vi "IMAQ FPGA Camera Link Pixel Packer U8x2.vi"(8 "Input Valid":bool, 9 "Frame Valid In":bool, 10 "Line Valid In":bool, 11 "Pixels In":u8[](array[numeric])=[0, 0]) -> (0 "Output Valid":bool, 1 "Frame Valid Out":bool, 2 "Line Valid Out":bool, 3 "Pixel Bus x8 Out":cluster{"Pixels":u8[], "DV":bool[]})   [LabVIEW 2017]
doc: "The Pixel Packer combines pixels from different cycles to create a Pixel Bus with 8 adjacent pixels. The DV flag in the Pixel Bus x8 Out indicates if the corresponding pixel is valid in case there are cameras with a width that is not a multiple of 8."
uses:
  <vilib>/visionFPGA/Basics/Camera Link Acquisition/Controls/IMAQ FPGA Camera Link Pixel Packer State.ctl
  <vilib>/visionFPGA/NI_VDM_FPGA_Basics.lvlib
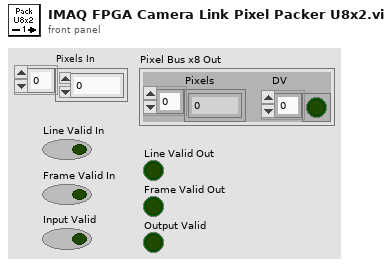
[diagram p1: front panel]
types:
  T1 = typedef "IMAQ FPGA Camera Link Pixel Packer State.ctl" = enum16{"Wait to Pack", "Pack", "Add EOL", "Check EOI"}
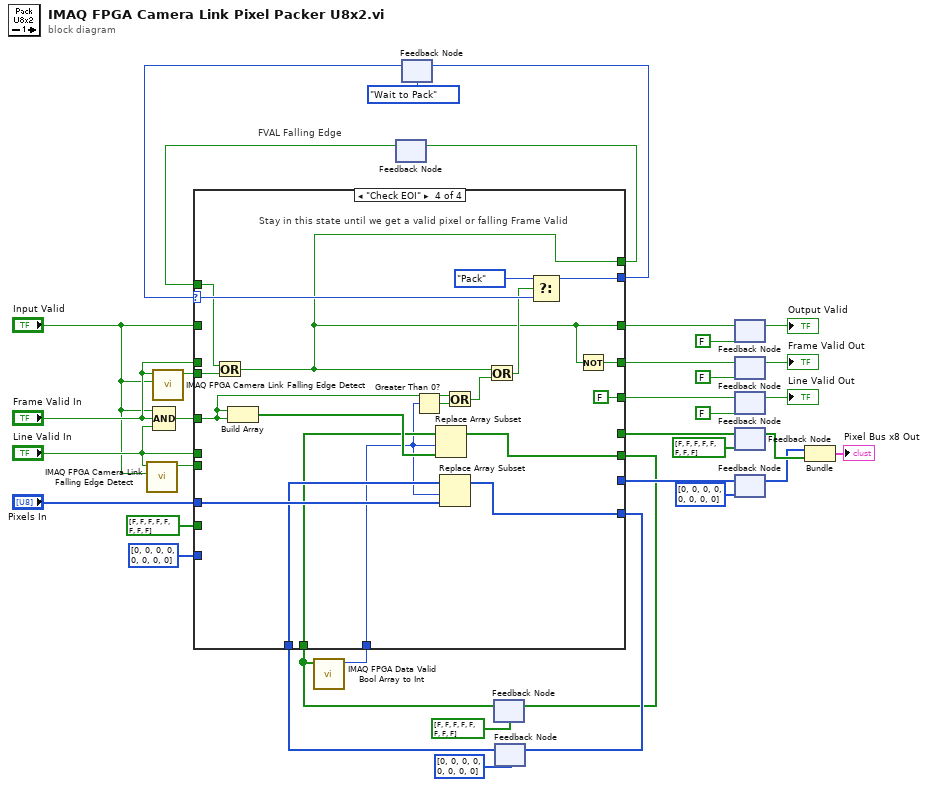
[diagram p0: block diagram]
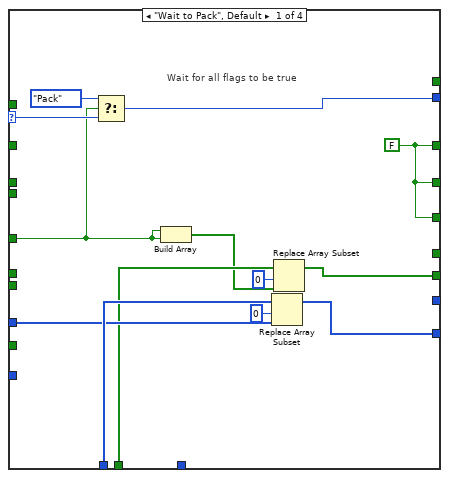
[diagram p2: hidden frame]
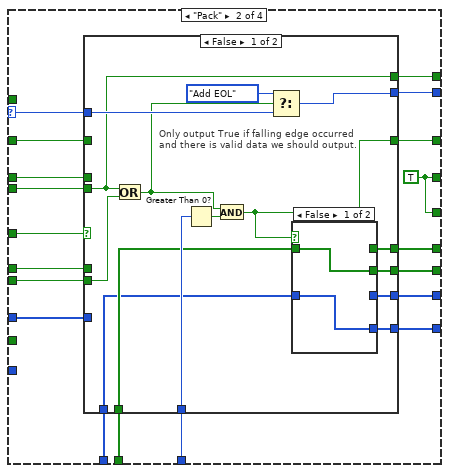
[diagram p3: hidden frame]
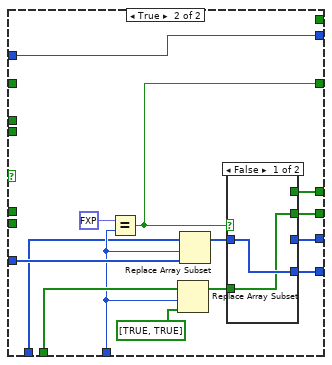
[diagram p5: hidden frame]
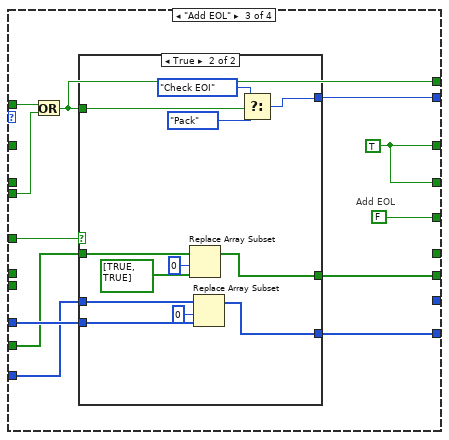
[diagram p7: hidden frame]
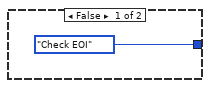
[diagram p8: hidden frame]
diagram:
  # "FVAL Falling Edge"
  n1 = call <vilib>:"IMAQ FPGA Camera Link Falling Edge Detect.vi"("Input Valid"="Input Valid", "Input"="Line Valid In") -> ("Falling Edge"=w7:bool)  [unwired: 9 in]
  n2 = call <vilib>:"IMAQ FPGA Camera Link Falling Edge Detect.vi"("Input Valid"="Input Valid", "Input"="Frame Valid In") -> ("Falling Edge"=w10:bool)  [unwired: 9 in]
  n3 = Compound Arithmetic op=AND("Input Valid", "Frame Valid In", "Line Valid In") -> (w16:bool)
  n4 = feedback #1() -> (w1:bool)  [unwired: 1 in]
  n5 = feedback #2(IMAQ_FPGA_Camera_Link_Pixel_Packer_State."Wait to Pack" ("Enum")) -> (w18:T1)
  n6 = feedback #3(bool[] [FALSE, FALSE, FALSE, FALSE, FALSE, FALSE, FALSE, FALSE]) -> (w4:bool[])
  n7 = call <vilib>:"IMAQ FPGA Data Valid Bool Array to Int.vi"("DV In"=w4) -> ("Sum DV Out"=w3:u8)  [unwired: 10 in]
  n8 = feedback #4(u8[] [0, 0, 0, 0, 0, 0, 0, 0] ("Pixels")) -> (w30:u8[])
  n9 = case shown="\"Check EOI\"" w18 {
    selector: w18 -> [w50 w68 _ w150]
    tunnel: w4 -> [w44 w56 _ w137]
    tunnel: w30 -> [w48 w67 _ w138]
    tunnel: [_ w64 _ _] -> w29
    tunnel: [_ w63 _ _] -> w22
    tunnel: [w38 w62 w118 w141] -> w36
    tunnel: [w38 w53 w118 w140] -> w20
    tunnel: [w38 w53 FALSE FALSE ("Frame Valid In")] -> w19
    tunnel: "Frame Valid In" -> [_ w60 _ _]
    tunnel: "Line Valid In" -> [_ w61 _ _]
    tunnel: "Input Valid" -> [_ w59 _ _]
    tunnel: w16 -> [w40 w69 w117 w134]
    tunnel: "Pixels In" -> [w46 w57 w114 w148]
    tunnel: [w45 w66 w113 w146] -> w14
    tunnel: [w42 w65 w115 w147] -> w13
    tunnel: [w41 w58 w116 w149] -> w12
    tunnel: w10 -> [_ w55 w108 w142]
    tunnel: w7 -> [_ w54 _ _]
    tunnel: u8[] [0, 0, 0, 0, 0, 0, 0, 0] ("Pixels") -> [_ _ w111 _]
    tunnel: bool[] [FALSE, FALSE, FALSE, FALSE, FALSE, FALSE, FALSE, FALSE] -> [_ _ w110 _]
    tunnel: w3 -> [_ w52 _ w136]
    tunnel: [_ w51 w107 w141] -> w2
    tunnel: w1 -> [_ _ w109 w143]
    frame "Wait to Pack", Default {
      w38 = FALSE
      # "Wait for all flags to be true"
      n10 = Select(t=IMAQ_FPGA_Camera_Link_Pixel_Packer_State."Pack", s=w40, f=w50) -> (s? t:f=w41:T1)
      n11 = Build Array(w40, w40) -> (w39:bool[])
      n12 = Replace Array Subset(array=w48, new element=w46, index=0) -> (w45:u8[])
      n13 = Replace Array Subset(array=w44, new element=w39, index=0) -> (w42:bool[])
    }
    frame "Pack" {
      w53 = TRUE ("Frame Valid In")
      n14 = case shown="False" w69 {
        tunnel: w68 -> [w83 w101]
        tunnel: [w81 w101] -> w58
        tunnel: w67 -> [w76 w94]
        tunnel: [w71 w91] -> w66
        tunnel: w56 -> [w77 w102]
        tunnel: [w72 w97] -> w65
        tunnel: [w74 w92] -> w64
        tunnel: [w75 w98] -> w63
        tunnel: w59 -> [_ _]
        tunnel: [w73 w100] -> w62
        tunnel: w60 -> [_ _]
        tunnel: w61 -> [_ _]
        tunnel: w55 -> [w70 _]
        tunnel: w54 -> [w84 _]
        tunnel: w52 -> [w80 w95]
        tunnel: w57 -> [_ w96]
        tunnel: [w70 _] -> w51
        frame False {
          # "Only output True if falling edge occurred and there is valid data we should output."
          n15 = Or(x=w70, y=w84) -> (x .or. y?=w78:bool)
          n16 = Greater Than 0?(x=w80) -> (x > 0?=w79:bool)
          n17 = And(x=w78, y=w79) -> (x .and. y?=w73:bool)
          n18 = Select(t=IMAQ_FPGA_Camera_Link_Pixel_Packer_State."Add EOL", s=w78, f=w83) -> (s? t:f=w81:T1)
          n19 = case shown="False" w73 {
            tunnel: w77 -> [w86 w88]
            tunnel: w76 -> [w85 w87]
            tunnel: [_ w88] -> w75
            tunnel: [_ w87] -> w74
            tunnel: [w86 _] -> w72
            tunnel: [w85 _] -> w71
            frame False {
            }
            frame True {
            }
          }
        }
        frame True {
          n20 = Equal?(x=fxp<+,4,4> 6.0, y=w95) -> (x = y?=w100:bool)
          n21 = Replace Array Subset(array=w102, new element=bool[] [TRUE, TRUE], index=w95) -> (w99:bool[])
          n22 = Replace Array Subset(array=w94, new element=w96, index=w95) -> (w93:u8[])
          n23 = case shown="False" w100 {
            tunnel: w99 -> [w103 w106]
            tunnel: [_ w106] -> w98
            tunnel: [w103 _] -> w97
            tunnel: w93 -> [w104 w105]
            tunnel: [_ w105] -> w92
            tunnel: [w104 _] -> w91
            frame False {
            }
            frame True {
            }
          }
        }
      }
    }
    frame "Add EOL" {
      w118 = TRUE
      # "Add EOL"
      n24 = Or(x=w109, y=w108) -> (x .or. y?=w107:bool)
      n25 = case shown="True" w117 {
        tunnel: [IMAQ_FPGA_Camera_Link_Pixel_Packer_State."Check EOI" ("Enum") w120] -> w116
        tunnel: w110 -> [_ w131]
        tunnel: [_ w130] -> w115
        tunnel: w111 -> [_ w129]
        tunnel: w114 -> [_ w128]
        tunnel: [_ w126] -> w113
        tunnel: w107 -> [_ w121]
        frame False {
        }
        frame True {
          n26 = Replace Array Subset(array=w131, new element=bool[] [TRUE, TRUE], index=0) -> (w130:bool[])
          n27 = Replace Array Subset(array=w129, new element=w128, index=0) -> (w126:u8[])
          n28 = Select(t=IMAQ_FPGA_Camera_Link_Pixel_Packer_State."Check EOI" ("Enum"), s=w121, f=IMAQ_FPGA_Camera_Link_Pixel_Packer_State."Pack" ("Enum")) -> (s? t:f=w120:T1)
        }
      }
    }
    frame "Check EOI" {
      # "Stay in this state until we get a valid pixel or falling Frame Valid"
      n29 = Or(x=w143, y=w142) -> (x .or. y?=w141:bool)
      n30 = Build Array(w134, w134) -> (w145:bool[])
      n31 = Greater Than 0?(x=w136) -> (x > 0?=w135:bool)
      n32 = Replace Array Subset(array=w137, new element=w145, index=w136) -> (w147:bool[])
      n33 = Replace Array Subset(array=w138, new element=w148, index=w136) -> (w146:u8[])
      n34 = Or(x=w134, y=w135) -> (x .or. y?=w132:bool)
      n35 = Or(x=w141, y=w132) -> (x .or. y?=w144:bool)
      n36 = Select(t=IMAQ_FPGA_Camera_Link_Pixel_Packer_State."Pack" ("Enum"), s=w144, f=w150) -> (s? t:f=w149:T1)
      n37 = Not(x=w141) -> (.not. x?=w140:bool)
    }
  }
  n38 = feedback-in #1(w2) -> ()
  n39 = feedback-in #2(w12) -> ()
  n40 = feedback-in #3(w13) -> ()
  n41 = feedback-in #4(w14) -> ()
  n42 = feedback #5(FALSE) -> (→"Output Valid":bool)
  n43 = feedback-in #5(w36) -> ()
  n44 = feedback #6(FALSE) -> (→"Frame Valid Out":bool)
  n45 = feedback-in #6(w20) -> ()
  n46 = feedback #7(FALSE) -> (→"Line Valid Out":bool)
  n47 = feedback-in #7(w19) -> ()
  n48 = feedback #8(bool[] [FALSE, FALSE, FALSE, FALSE, FALSE, FALSE, FALSE, FALSE]) -> (w27:bool[])
  n49 = feedback-in #8(w22) -> ()
  n50 = feedback #9(u8[] [0, 0, 0, 0, 0, 0, 0, 0] ("Pixels")) -> (w26:u8[])
  n51 = feedback-in #9(w29) -> ()
  n52 = Bundle("Pixels"=w26, w27) -> (→"Pixel Bus x8 Out":cluster{"Pixels":u8[], bool[]})  [unwired: 1 in]
